vi "参数初始化.vi"   [LabVIEW 2016]
types:
  T1 = typedef "数据库类型.ctl" = enum16{"Access", "SQLite"}
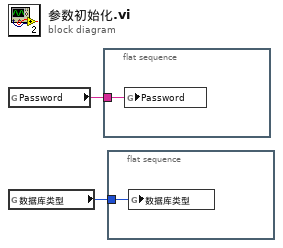
[diagram p0: block diagram]
diagram:
  n1 = global read "系统设置全局变量.vi" "Password"() -> (w1:string)
  n2 = global read "系统设置全局变量.vi" "数据库类型"() -> (w2:T1)
  n3 = flat-sequence {
    tunnel: w1 -> [w3]
    frame #0 {
      n4 = global write "外部调用接口全局变量.vi" "Password"(w3) -> ()
    }
  }
  n5 = flat-sequence {
    tunnel: w2 -> [w4]
    frame #0 {
      n6 = global write "外部调用接口全局变量.vi" "数据库类型"(w4) -> ()
    }
  }
